vi "Optionen Anzeige zum Speichern.vi"(7 "Optionen Anzeige (Eingang)":refnum<vi>, 8 "error in (no error)":errorcluster caption="Fehler (Eingang, kein Fehler)", 9 "Optionen fix":T1, 10 "sichtbar":bool[](array[boolean]), 11 "Optionen Anzeige (Eingang)":T2) -> (0 "error out":errorcluster caption="Fehler (Ausgang)", 3 "Optionen out":T1)   [LabVIEW 2020, in "System Einstellungen V2.lvlib"]
uses:
  System Einstellungen V2.lvlib
  Optionen Eingabe.ctl
  Visualisierungs Elemente/Checkbox(boolsch).ctl
  Optionen.ctl
  <vilib>/Utility/Data Type/NI_Data Type.lvlib
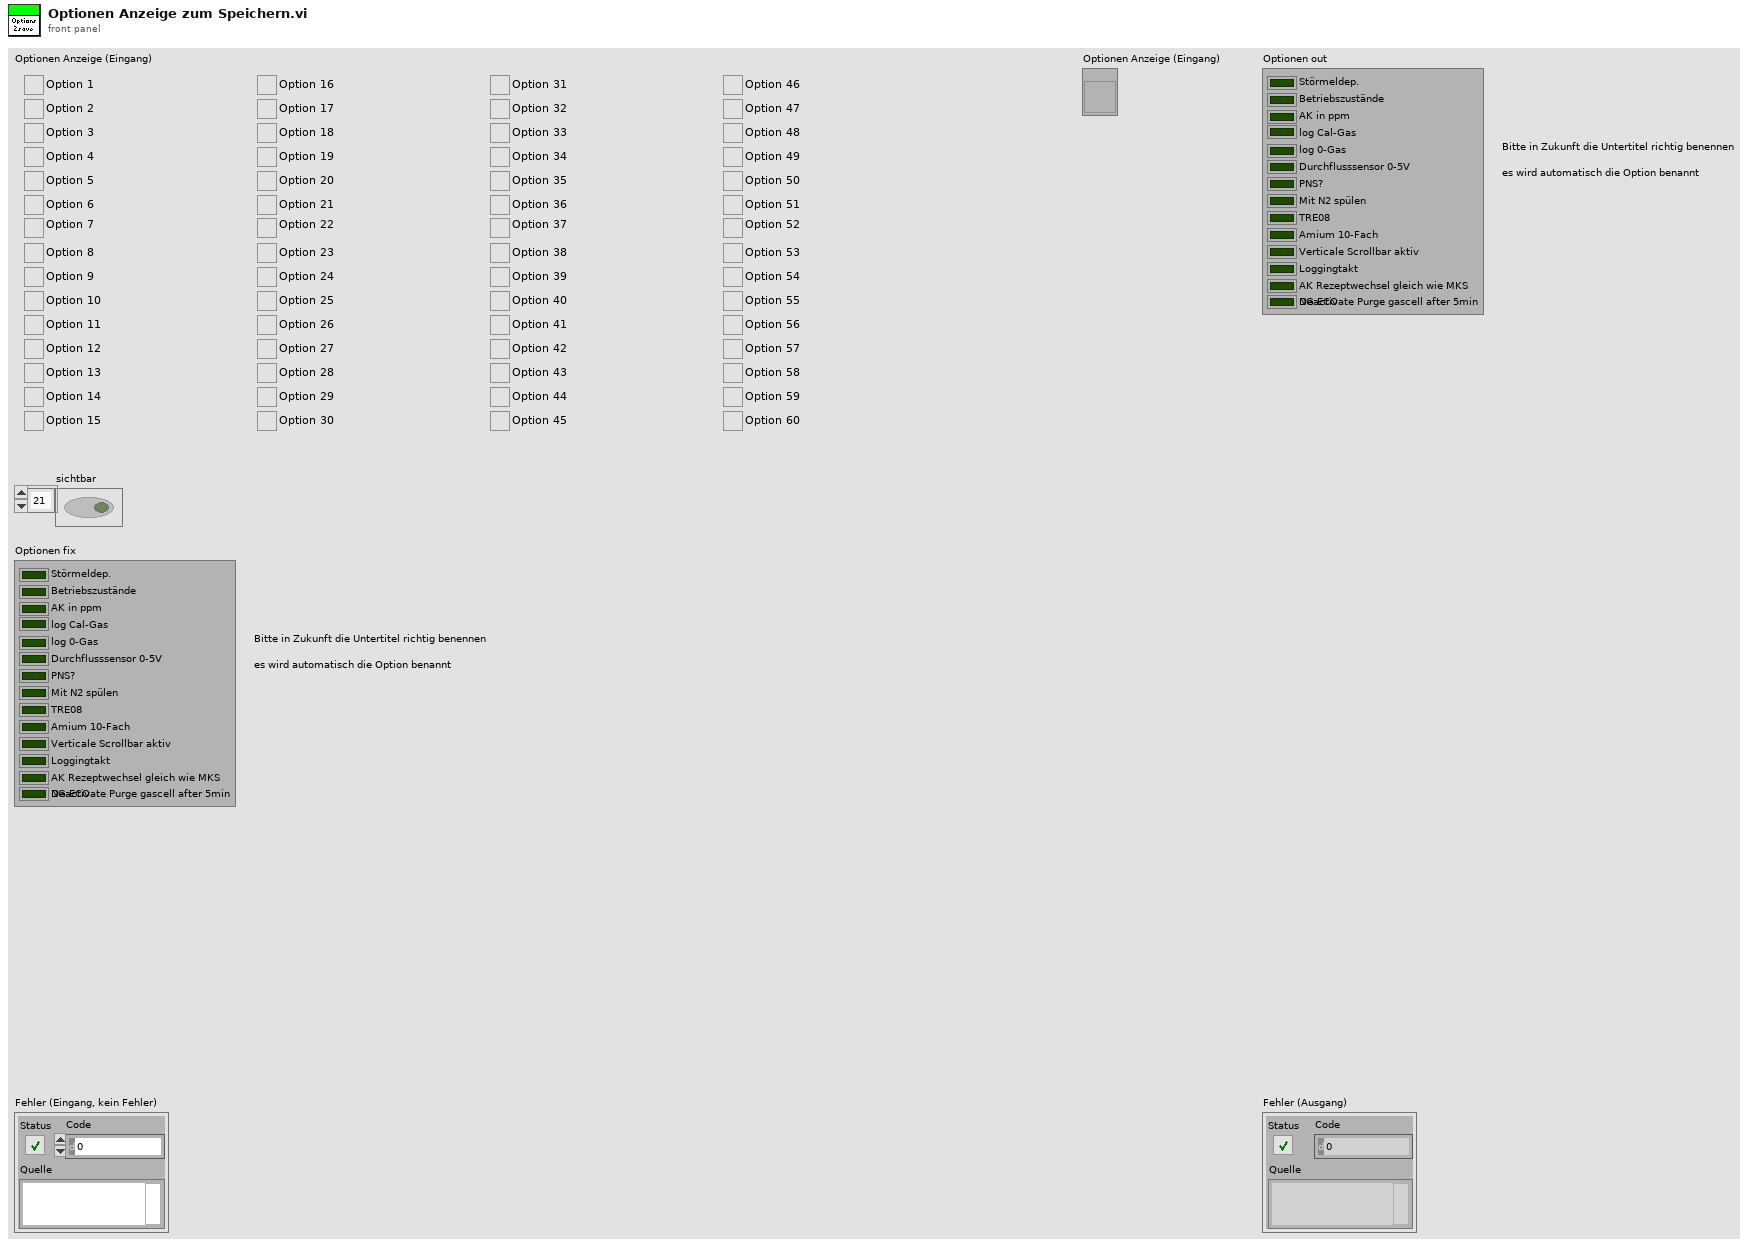
[diagram p1: front panel]
types:
  T1 = typedef "System Einstellungen V2.lvlib/Optionen.ctl" = cluster{"Störmeldep.":bool, "Betriebszustände":bool, "AK in ppm":bool, "log Cal-Gas":bool, "log 0-Gas":bool, "Durchflusssensor 0-5V":bool, "PNS?":bool, "Mit N2 spülen":bool, "TRE08":bool, "Amium 10-Fach":bool, "Verticale Scrollbar aktiv":bool, "Loggingtakt":bool, "AK Rezeptwechsel gleich wie MKS":bool, "NG ECO":bool}
  T2 = typedef "System Einstellungen V2.lvlib/Optionen Eingabe.ctl" = cluster{"Option 1":T3, "Option 2":T3, "Option 3":T3, "Option 4":T3, "Option 5":T3, "Option 6":T3, "Option 7":T3, "Option 8":T3, "Option 9":T3, "Option 10":T3, "Option 11":T3, "Option 12":T3, "Option 13":T3, "Option 14":T3, "Option 15":T3, "Option 16":T3, "Option 17":T3, "Option 18":T3, "Option 19":T3, "Option 20":T3, "Option 21":T3, "Option 22":T3, "Option 23":T3, "Option 24":T3, "Option 25":T3, "Option 26":T3, "Option 27":T3, "Option 28":T3, "Option 29":T3, "Option 30":T3, "Option 31":T3, "Option 32":T3, "Option 33":T3, "Option 34":T3, "Option 35":T3, "Option 36":T3, "Option 37":T3, "Option 38":T3, "Option 39":T3, "Option 40":T3, "Option 41":T3, "Option 42":T3, "Option 43":T3, "Option 44":T3, "Option 45":T3, "Option 46":T3, "Option 47":T3, "Option 48":T3, "Option 49":T3, "Option 50":T3, "Option 51":T3, "Option 52":T3, "Option 53":T3, "Option 54":T3, "Option 55":T3, "Option 56":T3, "Option 57":T3, "Option 58":T3, "Option 59":T3, "Option 60":T3}
  T3 = typedef "Checkbox(boolsch).ctl" = bool
  T4 = typedef "NI_Data Type.lvlib/Data Type.ctl" = enum8{"Invalid Type", "Void", "I8", "I16", "I32", "I64", "U8", "U16", "U32", "U64", "Single Float", "Double Float", "Extended Float", "Single Complex", "Double Complex", "Extended Complex", "Enum U8", "Enum U16", "Enum U32", "Enum U64", "Single Float With Unit", "Double Float With Unit", "Extended Float With Unit", "Single Complex with Unit", "Double Complex with Unit", "Extended Complex with Unit", "Boolean", "String", "Path", "Picture", "Tag", "Array", "Cluster", "Variant", "LV Variant", "Waveform", "Timestamp", "Digital Waveform", "Digital Data", "ExpressData", "Refnum", "External Data", "VI", "Poly VI", "LabVIEW Class Instance", "Fixed Point", "Set Collection", "Map Collection"}
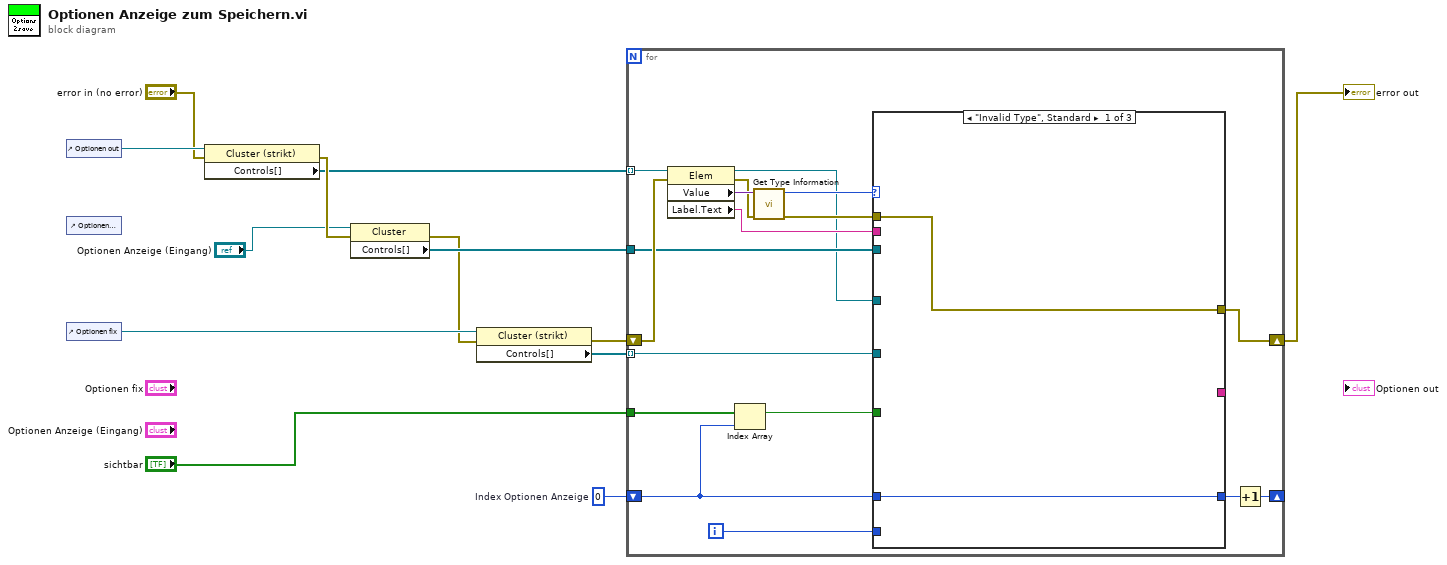
[diagram p0: block diagram]
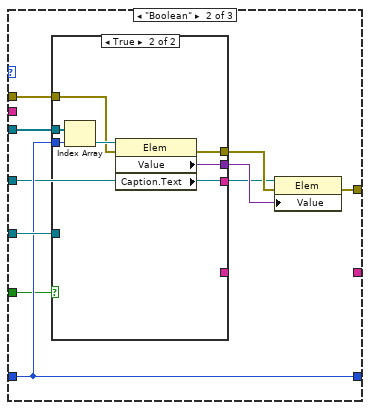
[diagram p2: hidden frame]
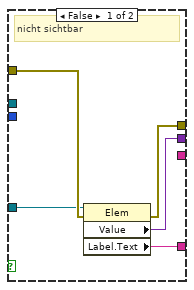
[diagram p3: hidden frame]
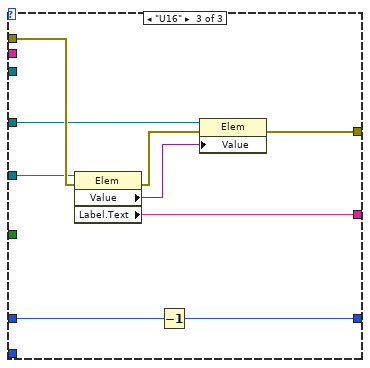
[diagram p4: hidden frame]
diagram:
  w3 = 0  # Index Optionen Anzeige
  n1 = control-ref of="Optionen out"() -> (w13:refnum<vi>)
  n2 = control-ref of="Optionen Anzeige (Eingang)"() -> ()  [unwired: 1 out]
  n3 = control-ref of="Optionen fix"() -> (w8:refnum<vi>)
  n4 = property class="Cluster (strikt)"(reference=w13, error in="error in (no error)") -> (error out=w11:errorcluster, "Controls[]"=w10:refnum<vi>[])  [unwired: 1 out]
  n5 = property class="Cluster"(reference="Optionen Anzeige (Eingang)", error in=w11) -> (error out=w6:errorcluster, "Controls[]"=w9:refnum<vi>[])  [unwired: 1 out]
  n6 = property class="Cluster (strikt)"(reference=w8, error in=w6) -> (error out=w5:errorcluster, "Controls[]"=w7:refnum<vi>[])  [unwired: 1 out]
  n7 = for {
    tunnel: w10 -> [w19] mode=indexing
    tunnel: w9 -> [w24]
    tunnel: w7 -> [w21] mode=indexing
    shift-right: [w20] -> w4
    shift-left: w5 -> [w30]
    shift-right: [w25] -> _
    shift-left: w3 -> [w17]
    tunnel: "sichtbar" -> [w22]
    i -> [w15]
    n8 = property class="Elem"(reference=w19, error in=w30) -> (reference out=w14:refnum<vi>, error out=w28:errorcluster, "Value"=w29:variant, "Label.Text"=w16:string)
    n9 = Index Array(array=w22, index=w17) -> (element=w18:bool)
    n10 = call <vilib>:"Get Type Information.vi"("error in (no error)"=w28, "variant"=w29) -> ("error out"=w23:errorcluster, "type"=w27:T4)  [unwired: 5 in, 3 out]
    n11 = case shown="\"Invalid Type\", Standard" w27 {
      tunnel: w17 -> [w32 w35 w61]
      tunnel: [w32 w35 w57] -> w26
      tunnel: w24 -> [_ w41 _]
      tunnel: w23 -> [w31 w37 w60]
      tunnel: w18 -> [_ w34 _]
      tunnel: w21 -> [_ w36 w56]
      tunnel: w14 -> [_ w33 w55]
      tunnel: [w31 w38 w62] -> w20
      tunnel: [_ _ w54] -> _
      tunnel: w16 -> [_ _ _]
      tunnel: w15 -> [_ _ _]
      frame "Invalid Type", Default {
      }
      frame "Boolean" {
        n12 = case shown="True" w34 {
          tunnel: w41 -> [_ w53]
          tunnel: [w44 w51] -> w40
          tunnel: [w45 w50] -> w39
          tunnel: w35 -> [_ w49]
          tunnel: w37 -> [w46 w48]
          tunnel: w36 -> [w43 _]
          tunnel: [_ w47] -> _
          tunnel: [w42 _] -> _
          frame False {
            # "nicht sichtbar"
            n13 = property class="Elem"(reference=w43, error in=w46) -> (error out=w44:errorcluster, "Value"=w45:variant, "Label.Text"=w42:string)  [unwired: 1 out]
          }
          frame True {
            n14 = Index Array(array=w53, index=w49) -> (element=w52:refnum<vi>)
            n15 = property class="Elem"(reference=w52, error in=w48) -> (error out=w51:errorcluster, "Value"=w50:variant, "Caption.Text"=w47:string)  [unwired: 1 out]
          }
        }
        n16 = property class="Elem"(reference=w33, error in=w40, "Value"=w39) -> (error out=w38:errorcluster)  [unwired: 1 out]
      }
      frame "U16" {
        n17 = property class="Elem"(reference=w56, error in=w60) -> (error out=w59:errorcluster, "Value"=w58:variant, "Label.Text"=w54:string)  [unwired: 1 out]
        n18 = Decrement(x=w61) -> (x-1=w57:i32)
        n19 = property class="Elem"(reference=w55, error in=w59, "Value"=w58) -> (error out=w62:errorcluster)  [unwired: 1 out]
      }
    }
    n20 = Increment(x=w26) -> (x+1=w25:i32)
  }
  "error out" <- w4
